vi "solar_msg Q Filter.vi"(8 "error in (no error)":errorcluster, 10 "MSGs to Filter (\"\"=None)":string[](array[string]), 11 "Queue in":refnum<queue>) -> (0 "error out":errorcluster, 3 "Queue out":refnum<queue>)   [LabVIEW 2018]
doc: "This filters messages in the queue. Filter messages using wildcards ('*'). Filters are case insensitive.\nEx. 'MyTarget:MyCMD' = '*:MyCMD', 'MyTarget:*', '*:*'"
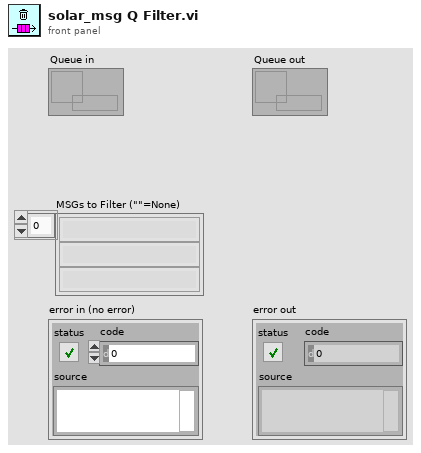
[diagram p1: front panel]
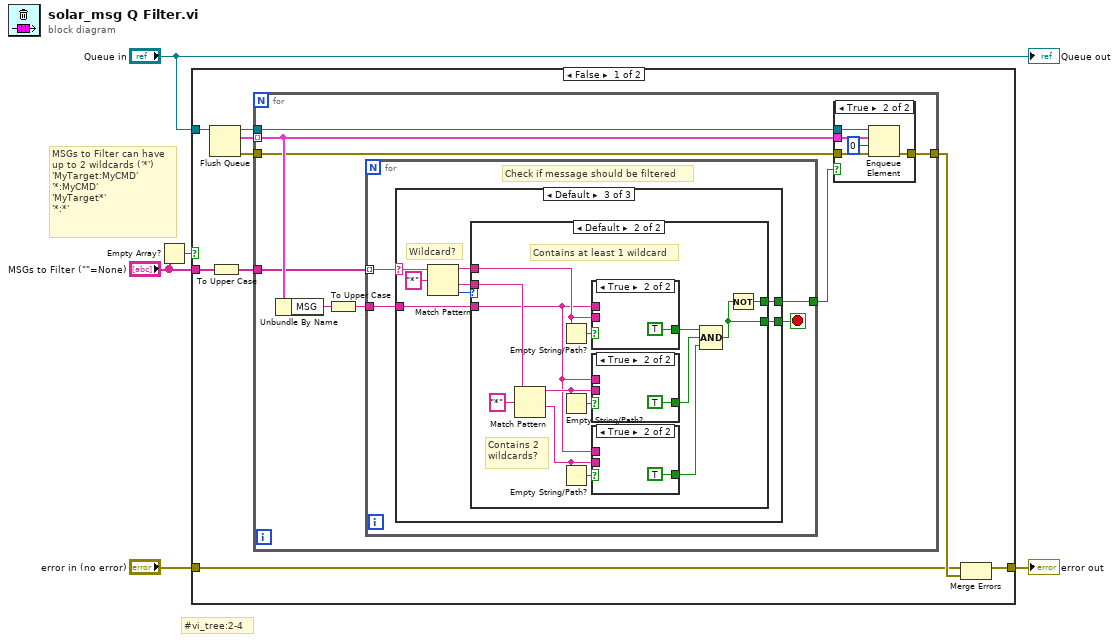
[diagram p0: block diagram]
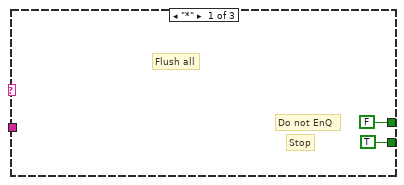
[diagram p3: hidden frame]
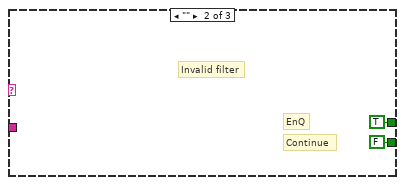
[diagram p4: hidden frame]
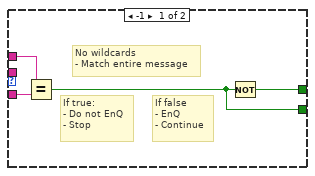
[diagram p5: hidden frame]
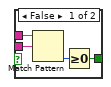
[diagram p6: hidden frame]
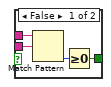
[diagram p7: hidden frame]
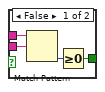
[diagram p8: hidden frame]
diagram:
  # "#vi_tree:2-4"
  # "MSGs to Filter can have\nup to 2 wildcards ('*')\n'MyTarget:MyCMD'\n'*:MyCMD'\n'MyTarget*'\n'*:*'"
  n1 = Empty Array?(array="MSGs to Filter (\"\"=None)") -> (empty?=w3:bool)
  n2 = case shown="False" w3 {
    tunnel: "Queue in" -> [w14 _]
    tunnel: "MSGs to Filter (\"\"=None)" -> [w11 _]
    tunnel: "error in (no error)" -> [w7 w78]
    tunnel: [w6 w78] -> w1
    frame False {
      n3 = Flush Queue(queue=w14) -> (queue out=w13:refnum<queue>, remaining elements=w12:cluster{"MSG":string, "DATA":variant}[], error out=w10:errorcluster)  [unwired: 1 in]
      n4 = To Upper Case(1:w11) -> (0:w9:string[])
      n5 = for {
        tunnel: w12 -> [w21] mode=indexing
        tunnel: w13 -> [w22]
        tunnel: w9 -> [w16]
        tunnel: w10 -> [w17]
        tunnel: [w15] -> w8
        n6 = Unbundle By Name(w21) -> ("MSG"=w19:string)
        n7 = To Upper Case(1:w19) -> (0:w20:string)
        n8 = for {
          tunnel: w16 -> [w31] mode=indexing
          tunnel: w20 -> [w32]
          tunnel: [w29] -> w18
          stop <- w30 stop-if-true
          # "Check if message should be filtered"
          n9 = case shown="Default" w31 {
            selector: w31 -> [_ _ w39]
            tunnel: w32 -> [_ _ w40]
            tunnel: [TRUE FALSE w38] -> w30
            tunnel: [FALSE TRUE w37] -> w29
            frame "*" {
              # "Stop"
              # "Do not EnQ"
              # "Flush all"
            }
            frame "" {
              # "EnQ"
              # "Continue"
              # "Invalid filter"
            }
            frame Default {
              # "Wildcard?"
              n10 = Match Pattern(string=w39, regular expression="*") -> (before substring=w42:string, after substring=w41:string, offset past match=w43:i32)  [unwired: 1 in, 1 out]
              n11 = case shown="Default" w43 {
                tunnel: w42 -> [w47 w62]
                tunnel: w41 -> [_ w57]
                tunnel: w40 -> [w48 w53]
                tunnel: [w46 w51] -> w38
                tunnel: [w45 w59] -> w37
                frame -1 {
                  # "If false\n- EnQ\n- Continue"
                  # "If true:\n- Do not EnQ\n- Stop"
                  # "No wildcards\n- Match entire message"
                  n12 = Equal?(x=w47, y=w48) -> (x = y?=w46:bool)
                  n13 = Not(x=w46) -> (.not. x?=w45:bool)
                }
                frame Default {
                  # "Contains 2 \nwildcards?"
                  # "Contains at least 1 wildcard"
                  n14 = Match Pattern(string=w57, regular expression="*") -> (before substring=w56:string, after substring=w54:string)  [unwired: 1 in, 2 out]
                  n15 = Empty String/Path?(string/path=w62) -> (empty?=w61:bool)
                  n16 = Empty String/Path?(string/path=w56) -> (empty?=w60:bool)
                  n17 = Empty String/Path?(string/path=w54) -> (empty?=w55:bool)
                  n18 = case shown="True" w61 {
                    tunnel: w62 -> [w76 _]
                    tunnel: w53 -> [w75 _]
                    tunnel: [w73 TRUE] -> w52
                    frame False {
                      n19 = Match Pattern(string=w75, regular expression=w76) -> (offset past match=w74:i32)  [unwired: 1 in, 3 out]
                      n20 = Greater Or Equal To 0?(x=w74) -> (x >= 0?=w73:bool)
                    }
                    frame True {
                    }
                  }
                  n21 = case shown="True" w60 {
                    tunnel: w56 -> [w71 _]
                    tunnel: w53 -> [w70 _]
                    tunnel: [w68 TRUE] -> w50
                    frame False {
                      n22 = Match Pattern(string=w70, regular expression=w71) -> (offset past match=w69:i32)  [unwired: 1 in, 3 out]
                      n23 = Greater Or Equal To 0?(x=w69) -> (x >= 0?=w68:bool)
                    }
                    frame True {
                    }
                  }
                  n24 = case shown="True" w55 {
                    tunnel: w54 -> [w66 _]
                    tunnel: w53 -> [w65 _]
                    tunnel: [w63 TRUE] -> w49
                    frame False {
                      n25 = Match Pattern(string=w65, regular expression=w66) -> (offset past match=w64:i32)  [unwired: 1 in, 3 out]
                      n26 = Greater Or Equal To 0?(x=w64) -> (x >= 0?=w63:bool)
                    }
                    frame True {
                    }
                  }
                  n27 = Compound Arithmetic op=AND(w52, w50, w49) -> (w51:bool)
                  n28 = Not(x=w51) -> (.not. x?=w59:bool)
                }
              }
            }
          }
        }
        n29 = case shown="True" w18 {
          tunnel: w22 -> [_ w28]
          tunnel: w21 -> [_ w27]
          tunnel: w17 -> [w23 w25]
          tunnel: [w23 w24] -> w15
          frame False {
          }
          frame True {
            n30 = Enqueue Element(queue=w28, element=w27, timeout in ms (-1)=0, error in (no error)=w25) -> (error out=w24:errorcluster)  [unwired: 2 out]
          }
        }
      }
      n31 = Merge Errors(w7, w8) -> (w6:errorcluster)
    }
    frame True {
    }
  }
  "error out" <- w1
  "Queue out" <- "Queue in"
